vi "colormap_maker.vi"() -> ()   [LabVIEW 2014]
uses:
  <vilib>/Analysis/NI_AALBase.lvlib
  <vilib>/Analysis/1siggen.llb/Ramp Pattern by Samples.vi
  <vilib>/vision/NI_Vision_Development_Module.lvlib
panel:
  out "Waveform Graph":u16[][](graph)
  in  "Save color map":bool
  in  "max_number":dbl=255.0 caption="Maximum number"
  in  "min_number":dbl caption="Minimum number"
  in  "stop":bool
  in  "values_colors":cluster{dbl, u32}[](array[cluster])
  in  "q_colors":u32=2 caption="Quantity of colors" min=2
  out "Intensity Graph":dbl[][](graph)
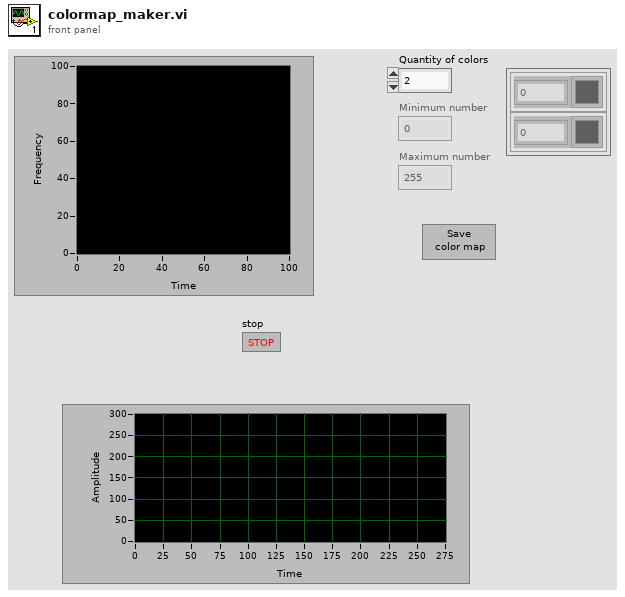
[diagram p1: front panel]
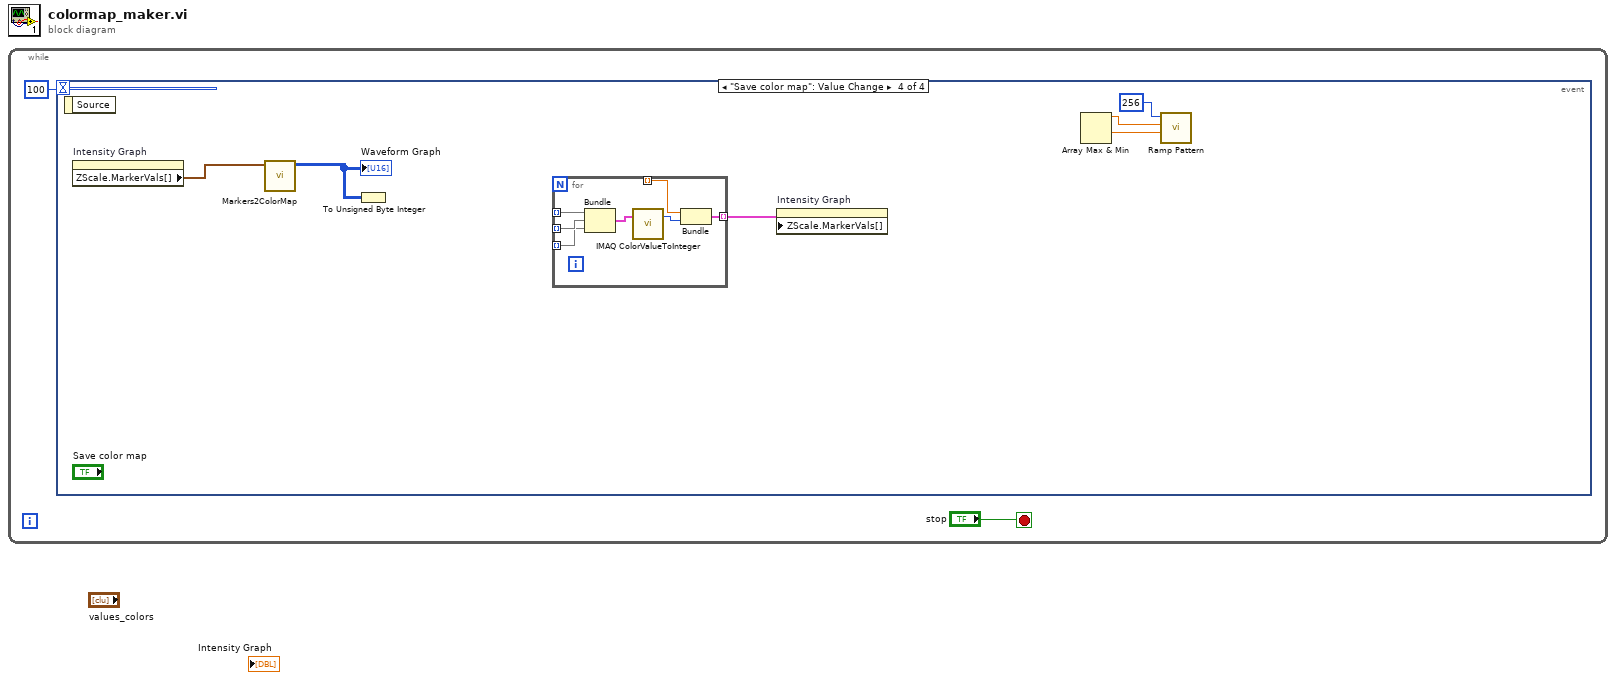
[diagram p0: block diagram]
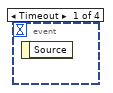
[diagram p2: hidden frame]
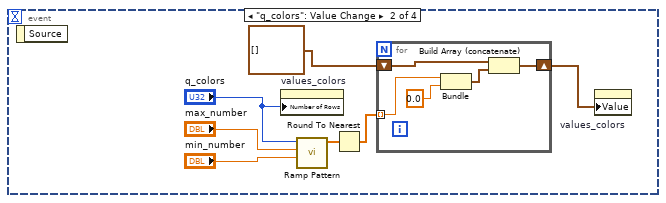
[diagram p3: hidden frame]
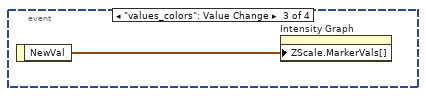
[diagram p4: hidden frame]
diagram:
  n1 = while {
    stop <- "stop" stop-if-true
    n2 = event shown="[3] \"Save color map\": Value Change" {
      selector: _ -> [_ _ _ _]
      dyn-events: _ -> [_ _ _ _]
      timeout: 100 -> [_ _ _ _]
      event Timeout {
        n3 = event-data() -> ()  [unwired: 1 in, 1 out]
      }
      event "q_colors": Value Change {
        n4 = event-data() -> ()  [unwired: 1 in, 1 out]
        n5 = property on="values_colors" class="Arr (strict)"("Number of Rows"="q_colors") -> ()  [unwired: 2 in, 2 out]
        n6 = call-poly <vilib>:"Ramp Pattern.vi"("start"="min_number", "end"="max_number", "samples"="q_colors") -> ("Ramp Pattern"=w7:dbl[])  [unwired: 7 in, 1 out]
        n7 = Round To Nearest(number=w7) -> (nearest integer value=w3:dbl[])
        n8 = for {
          tunnel: w3 -> [w11] mode=indexing
          shift-right: [w14] -> w5
          shift-left: cluster{"value":dbl, "color":dbl}[] [] -> [w13]
          n9 = Bundle(w11, 0.0) -> (w12:cluster{dbl, dbl})  [unwired: 1 in]
          n10 = Build Array (concatenate)(w13, w12) -> (w14:cluster{"value":dbl, "color":dbl}[])
        }
        n11 = property on="values_colors" class="Arr (strict)"("Value"=w5) -> ()  [unwired: 2 in, 2 out]
      }
      event "values_colors": Value Change {
        n12 = event-data() -> ("NewVal"=w15:cluster{dbl, u32}[])  [unwired: 1 in]
        n13 = property on="Intensity Graph" class="IntGraph (strict)"("ZScale.MarkerVals[]"=w15) -> ()  [unwired: 2 in, 2 out]
      }
      event "Save color map": Value Change {
        n14 = event-data() -> ()  [unwired: 1 in, 1 out]
        n15 = property on="Intensity Graph" class="IntGraph (strict)"() -> ("ZScale.MarkerVals[]"=w23:cluster{dbl, u32}[])  [unwired: 2 in, 2 out]
        n16 = call "Markers2ColorMap.vi"("Markers-colors"=w23) -> ("ColorMap"=w16:u16[][])  [unwired: 10 in]
        "Waveform Graph" <- w16
        n17 = To Unsigned Byte Integer(number=w16) -> ()  [unwired: 1 out]
        n18 = for {
          tunnel: _ -> [w30] mode=indexing
          tunnel: _ -> [w29] mode=indexing
          tunnel: _ -> [w28] mode=indexing
          tunnel: _ -> [w25] mode=indexing
          tunnel: [w24] -> w18 mode=indexing
          n19 = Bundle(w30, w29, w28) -> (w27:cluster{void, void, void})  [unwired: 1 in]
          n20 = call "IMAQ ColorValueToInteger"("Color Value"=w27) -> ("U32 value"=w26:u32)  [unwired: 4 in, 3 out]
          n21 = Bundle(w25, "U32 value"=w26) -> (w24:cluster{void, "U32 value":u32})  [unwired: 1 in]
        }
        n22 = property on="Intensity Graph" class="IntGraph (strict)"("ZScale.MarkerVals[]"=w18) -> ()  [unwired: 2 in, 2 out]
        n23 = Array Max & Min() -> (array=w17:dbl[], max value=w21:dbl, min value=w22:dbl)  [unwired: 2 out]
        n24 = call-poly <vilib>:"Ramp Pattern.vi"("start"=w22, "end"=w21, "samples"=256) -> ("Ramp Pattern"=w19:dbl[])  [unwired: 7 in, 1 out]
      }
    }
  }
